vi "Create.vi"(5 "Source Port":refnum<class "FSM.Port.lvclass">, 7 "Target Port":refnum<class "FSM.Port.lvclass">, 11 "edgeSpec":string) -> (4 "New Edge":refnum<class "FSM.Edge.lvclass">)   [LabVIEW 2020, in "FSM.Edge.lvclass"]
uses:
  FSM.Edge.lvclass
  FSM.Port/FSM.Port.lvclass
  FSM.EdgeEnd/EndStyle.ctl
  FSM.Port/FSM.Port.lvclass/FSM.Port.ctl
  FSM.Edge.lvclass/FSM.Edge.ctl
  FSM.Port/Read belongsTo.vi
  FSM.Port/Read Location.vi
  <vilib>/regexp/Match Regular Expression.xnode
  FSM.Label/FSM.Label.lvclass
  FSM.EdgeEnd/FSM.EdgeEnd.lvclass
  FSM.Annotation/FSM.Annotation.lvclass
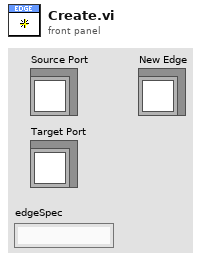
[diagram p1: front panel]
types:
  T1 = typedef "FSM.EdgeEnd.lvclass/EndStyle.ctl" = enum16{"Plain", "Arrow", "Box", "Circle", "Diamond"}
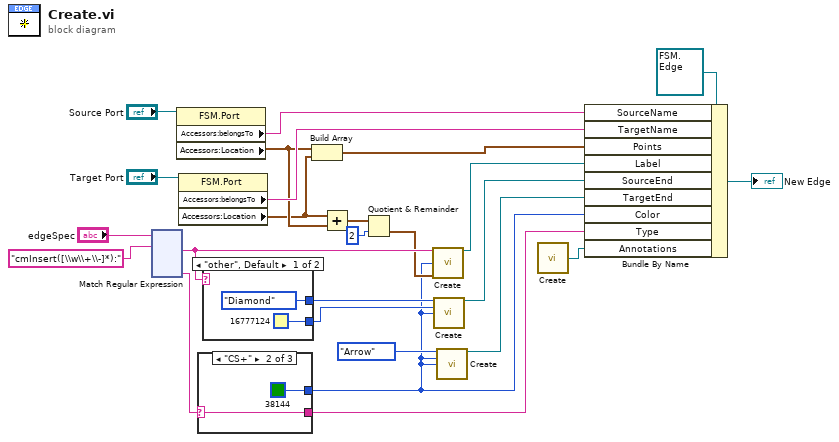
[diagram p0: block diagram]
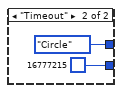
[diagram p2: hidden frame]
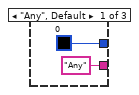
[diagram p3: hidden frame]
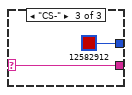
[diagram p4: hidden frame]
diagram:
  n1 = xnode "Match Regular Expression"("input string"="edgeSpec", "regular expression"="cmInsert([\\w\\+\\-]*):") -> ("after match"=w12:string, "submatch 1"=w4:string)  [unwired: 4 in, 4 out]
  n2 = property class="FSM.Port"(reference="Source Port") -> ("Accessors:belongsTo"=w22:string, "Accessors:Location"=w9:cluster{"x":i16, "y":i16})  [unwired: 1 in, 2 out]
  n3 = property class="FSM.Port"(reference="Target Port") -> ("Accessors:belongsTo"=w20:string, "Accessors:Location"=w8:cluster{"x":i16, "y":i16})  [unwired: 1 in, 2 out]
  n4 = case shown="\"CS+\"" w4 {
    selector: w4 -> [_ w28 w30]
    tunnel: [u32 0 u32 38144 u32 12582912] -> w2
    tunnel: ["Any" w28 w30] -> w3
    frame "Any", Default {
    }
    frame "CS+" {
    }
    frame "CS-" {
    }
  }
  n5 = case shown="\"other\", Default" w12 {
    tunnel: [EndStyle."Diamond" ("Serialized.EndStyle") EndStyle."Circle" ("Serialized.EndStyle")] -> w11
    tunnel: [u32 16777124 u32 16777215] -> w10
    frame "other", Default {
    }
    frame "Timeout" {
    }
  }
  n6 = Build Array(w9, w8) -> (w19:cluster{"x":i16, "y":i16}[])
  n7 = Add(x=w8, y=w9) -> (x+y=w7:cluster{"x":i16, "y":i16})
  n8 = Quotient & Remainder(x=w7, y=2) -> (floor(x/y)=w5:cluster{"x":i32, "y":i32})  [unwired: 1 out]
  n9 = call "Create.vi"("Serialized.Text"=w12, "Serialized.Color"=w2, "Serialized.Location"=w5) -> ("FSM.Label"=w18:refnum<class "FSM.Label.lvclass">)  [unwired: 12 in]
  n10 = call "Create.vi"("Serialized.EndStyle"=w11, "Serialized.FillColor"=w10, "Serialized.LineColor"=w2) -> ("output cluster"=w15:refnum<class "FSM.EdgeEnd.lvclass">)  [unwired: 12 in]
  n11 = call "Create.vi"("Serialized.EndStyle"=EndStyle."Arrow", "Serialized.FillColor"=w2, "Serialized.LineColor"=w2) -> ("output cluster"=w14:refnum<class "FSM.EdgeEnd.lvclass">)  [unwired: 12 in]
  n12 = call "Create.vi"() -> ("FSM.Annotation"=w1:refnum<class "FSM.Annotation.lvclass">)  [unwired: 15 in]
  n13 = Bundle By Name(cluster=refnum<class "FSM.Edge.lvclass"> refnum ("FSM.Edge"), "SourceName"=w22, "TargetName"=w20, "Points"=w19, "Label"=w18, "SourceEnd"=w15, "TargetEnd"=w14, "Color"=w2, "Type"=w3, "Annotations"=w1) -> (→"New Edge":refnum<class "FSM.Edge.lvclass">)
